vi "test Add State.vi"(8 "error in (no error)":errorcluster, 11 "TestCase in":refnum<class "Switch Scripting Unit Tests.lvclass">) -> (0 "error out":errorcluster, 3 "TestCase out":refnum<class "Switch Scripting Unit Tests.lvclass">)   [LabVIEW 2017, in "Switch Scripting Unit Tests.lvclass"]
uses:
  Switch Scripting Unit Tests.lvclass
  Shared/Routing State.ctl
  Shared/Connection.ctl
  Switch Scripting Unit Tests.lvclass/Switch Scripting Unit Tests.ctl
  <vilib>/addons/_JKI Toolkits/VI Tester/TestCase.llb/TestCase.lvclass
  Switch Scripting.lvlib
  Shared/Routing and Faulting Shared.lvlib
  C:/Program Files (x86)/National Instruments/LabVIEW 2017/vi.lib/addons/_JKI Toolkits/VI Tester/TestCase.llb/TestCase.lvclass
panel:
  in  "Save?":bool
  out "Output Filename":string
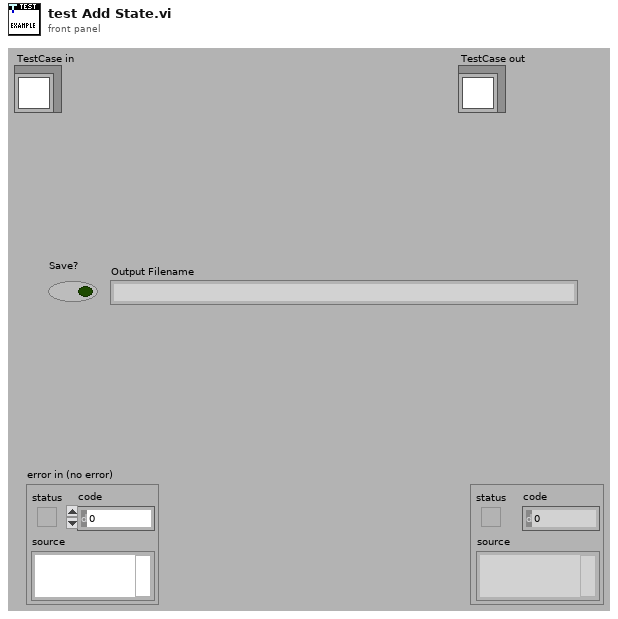
[diagram p1: front panel]
types:
  T1 = typedef "Routing and Faulting Shared.lvlib/Connection.ctl" = cluster{"Source":string, "Destination":string}
  T2 = typedef "Routing and Faulting Shared.lvlib/Routing State.ctl" = cluster{"Name":string, "Description":string, "Value":i32, "Connection List":T1[]}
  T3 = typedef "Custom Device API.lvlib/Custom Device Item Ref.ctl" = u64
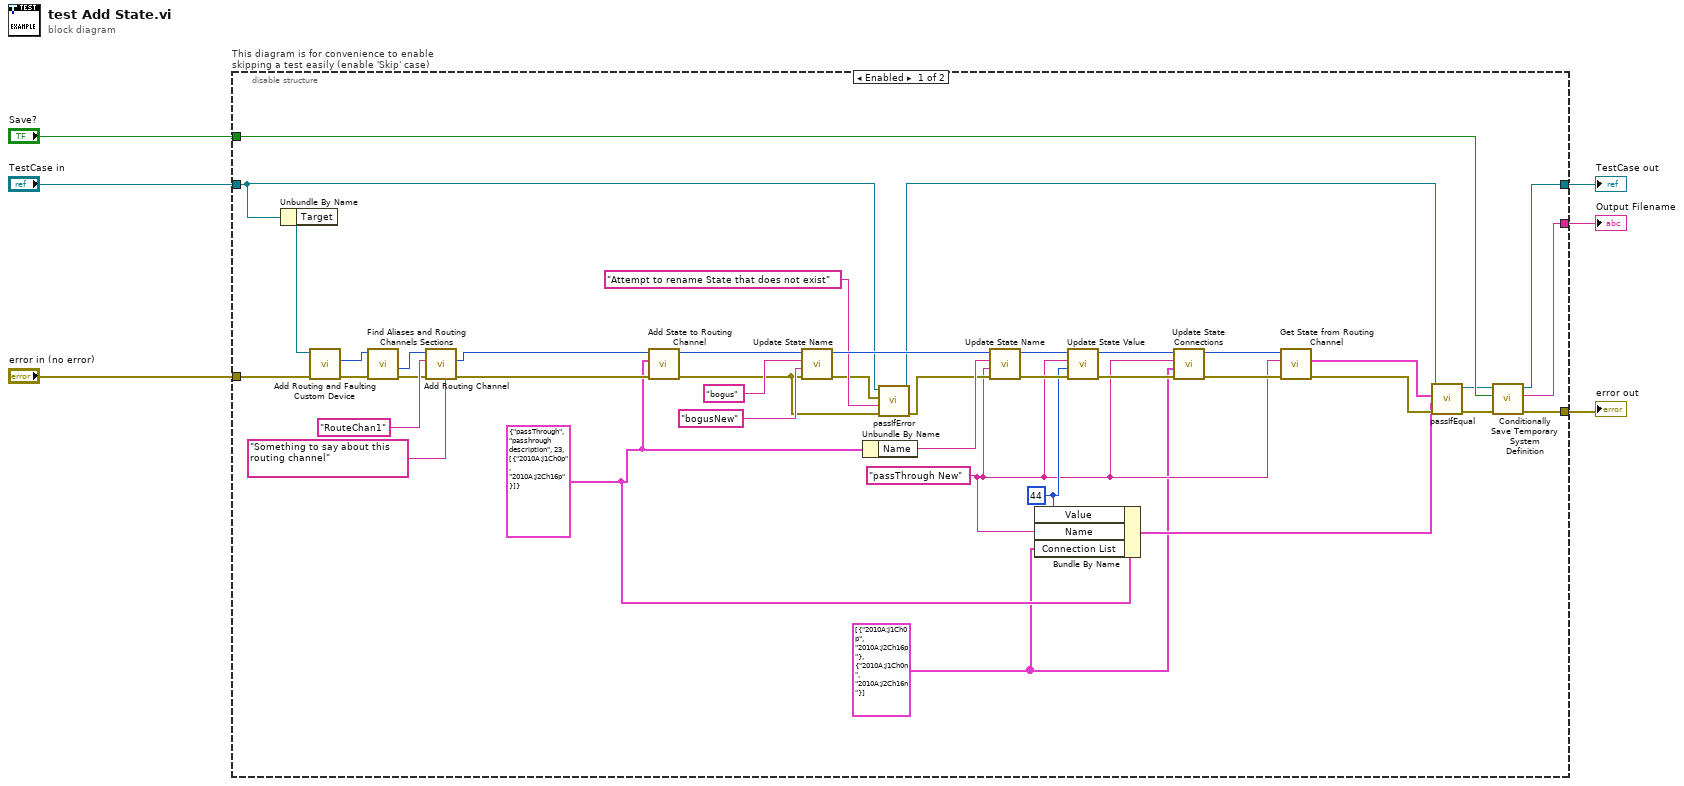
[diagram p0: block diagram]
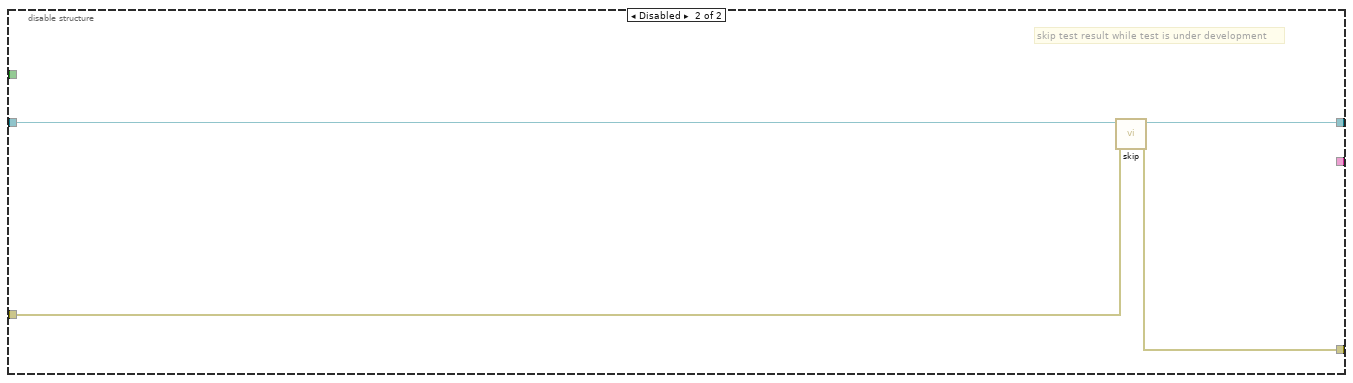
[diagram p2: hidden frame]
diagram:
  n1 = disable-structure "This diagram is for convenience to enable skipping a test easily (enable 'Skip' case)" shown="Enabled" {
    disable-tunnel: "TestCase in" -> [w20 w50]
    disable-tunnel: [w41 w48] -> w3
    disable-tunnel: [w45 w49] -> w5
    disable-tunnel: "error in (no error)" -> [w46 w47]
    disable-tunnel: [w44 _] -> w2
    disable-tunnel: "Save?" -> [w43 _]
    frame Enabled {
      w11 = T1[] [{"Source"="2010A:J1Ch0p", "Destination"="2010A:J2Ch16p"}, {"Source"="2010A:J1Ch0n", "Destination"="2010A:J2Ch16n"}] ("connection list")
      w30 = 44 ("New Value")
      w12 = "passThrough New" ("New State")
      w31 = T2 {"Name"="passThrough", "Description"="passhrough description", "Value"=23, "Connection List"=[{"Source"="2010A:J1Ch0p", "Destination"="2010A:J2Ch16p"}]} ("Routing State")
      n2 = Unbundle By Name(w20) -> ("Target"=w42:refnum<k24>)
      n3 = call "Add Routing and Faulting Custom Device.vi"("error in (no error)"=w46, "Target in"=w42) -> ("error out"=w40:errorcluster, "Routing and Faulting Custom Device Ref"=w9:T3)  [unwired: 7 in, 1 out]
      n4 = call "Find Aliases and Routing Channels Sections.vi"("error in (no error)"=w40, "Routing and Faulting Custom Device Ref in"=w9) -> ("error out"=w10:errorcluster, "Routing Channels Ref"=w8:T3)  [unwired: 6 in, 2 out]
      n5 = call "Add Routing Channel.vi"("Description"="Something to say about this routing channel", "error in (no error)"=w10, "Channel Name"="RouteChan1", "Routing Channels Ref in"=w8) -> ("error out"=w36:errorcluster, "Channel Ref"=w35:T3)  [unwired: 5 in, 1 out]
      n6 = call "Add State to Routing Channel.vi"("error in (no error)"=w36, "Routing Chanel State"=w31, "Channel Ref in"=w35) -> ("error out"=w24:errorcluster, "Channel Ref out"=w28:T3)  [unwired: 7 in]
      n7 = call "Update State Name.vi"("error in (no error)"=w24, "New State"="bogusNew" ("State"), "State"="bogus", "Channel Ref in"=w28) -> ("error out"=w22:errorcluster, "Channel Ref out"=w27:T3)  [unwired: 6 in]
      n8 = Unbundle By Name(w31) -> ("Name"=w34:string)
      n9 = call-dynamic "passIfError.vi"("error in (no error)"=w24, "task (\"\")"="Attempt to rename State that does not exist" ("custom report message (\"\")"), "error"=w22, "TestCase in"=w20) -> ("error out"=w21:errorcluster, "TestCase out"=w19:refnum<class "Switch Scripting Unit Tests.lvclass">)  [unwired: 6 in]
      n10 = call "Update State Name.vi"("error in (no error)"=w21, "New State"=w12, "State"=w34, "Channel Ref in"=w27) -> ("error out"=w32:errorcluster, "Channel Ref out"=w33:T3)  [unwired: 6 in]
      n11 = Bundle By Name(cluster=w31, "Value"=w30, "Name"=w12, "Connection List"=w11) -> (w17:T2)
      n12 = call "Update State Value.vi"("error in (no error)"=w32, "New Value"=w30, "State"=w12, "Channel Ref in"=w33) -> ("error out"=w16:errorcluster, "Channel Ref out"=w14:T3)  [unwired: 6 in]
      n13 = call "Update State Connections.vi"("error in (no error)"=w16, "Connection List"=w11, "State"=w12, "Channel Ref in"=w14) -> ("error out"=w15:errorcluster, "Channel Ref out"=w13:T3)  [unwired: 6 in]
      n14 = call "Get State from Routing Channel.vi"("error in (no error)"=w15, "State"=w12, "Channel Ref in"=w13) -> ("error out"=w29:errorcluster, "Routing Channel State"=w18:T2)  [unwired: 6 in, 1 out]
      n15 = call-dynamic "passIfEqual.vi"("error in (no error)"=w29, "y"=w17, "x"=w18, "TestCase in"=w19) -> ("error out"=w39:errorcluster, "TestCase out"=w38:refnum<class "Switch Scripting Unit Tests.lvclass">)  [unwired: 6 in]
      n16 = call "Conditionally Save Temporary System Definition.vi"("error in (no error)"=w39, "Save?"=w43, "Test Case"=w38) -> ("error out"=w45:errorcluster, "filename"=w44:string, "Test Case"=w41:refnum<class "Switch Scripting Unit Tests.lvclass">)  [unwired: 6 in]
    }
    frame Disabled {
      # "skip test result while test is under development"
      n17 = call <vilib>:"skip.vi"("error in (no error)"=w47, "TestCase in"=w50) -> ("error out"=w49:errorcluster, "TestCase out"=w48:refnum<class "Switch Scripting Unit Tests.lvclass">)  [unwired: 8 in]
    }
  }
  "error out" <- w5
  "TestCase out" <- w3
  "Output Filename" <- w2
